vi "GetData.vi"(7 "LabVIEW Web Service Request":refnum<class "Web Request.lvclass">) -> (0 "Ball":T1, 1 "Corners":cluster{"X":sgl, "Y":sgl}[](array[cluster]), 2 "Red Team Data":T2, 3 "Blue Team Data":T2)   [LabVIEW 2018]
uses:
  <vilib>/wsapi/Web Request.lvclass
  Ball Data.vi
  Blue Team Data.vi
  Red Team Data.vi
  Table Data.vi
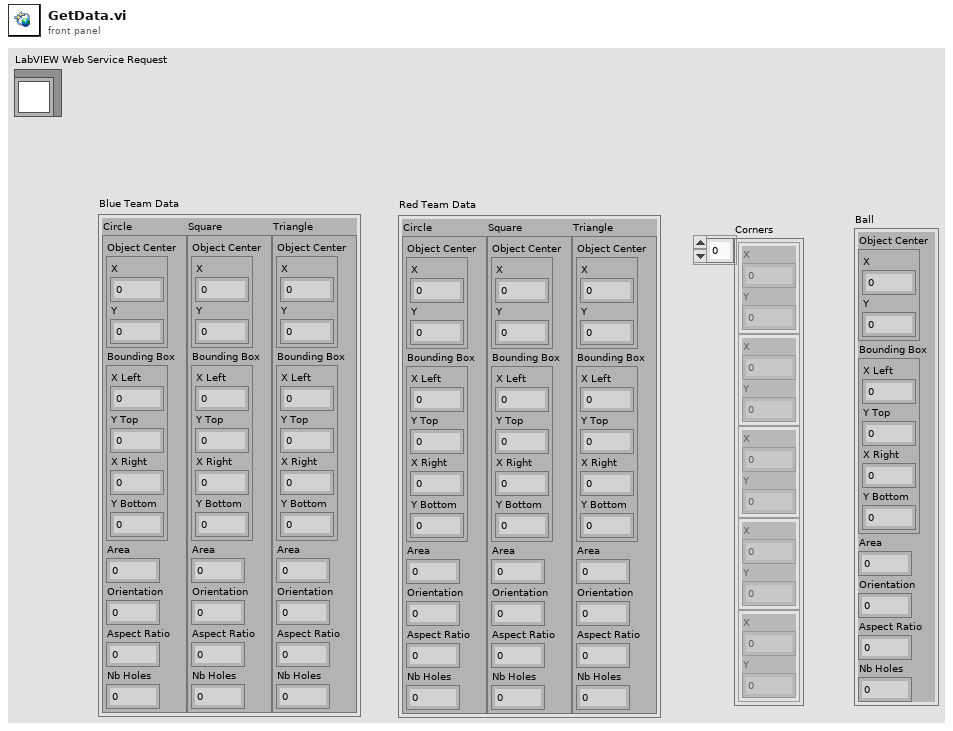
[diagram p1: front panel]
types:
  T1 = cluster{"Object Center":cluster{"X":sgl, "Y":sgl}, "Bounding Box":cluster{"X Left":i32, "Y Top":i32, "X Right":i32, "Y Bottom":i32}, "Area":sgl, "Orientation":sgl, "Aspect Ratio":sgl, "Nb Holes":i32}
  T2 = cluster{"Circle":cluster{"Object Center":cluster{"X":sgl, "Y":sgl}, "Bounding Box":cluster{"X Left":i32, "Y Top":i32, "X Right":i32, "Y Bottom":i32}, "Area":sgl, "Orientation":sgl, "Aspect Ratio":sgl, "Nb Holes":i32}, "Square":cluster{"Object Center":cluster{"X":sgl, "Y":sgl}, "Bounding Box":cluster{"X Left":i32, "Y Top":i32, "X Right":i32, "Y Bottom":i32}, "Area":sgl, "Orientation":sgl, "Aspect Ratio":sgl, "Nb Holes":i32}, "Triangle":cluster{"Object Center":cluster{"X":sgl, "Y":sgl}, "Bounding Box":cluster{"X Left":i32, "Y Top":i32, "X Right":i32, "Y Bottom":i32}, "Area":sgl, "Orientation":sgl, "Aspect Ratio":sgl, "Nb Holes":i32}}
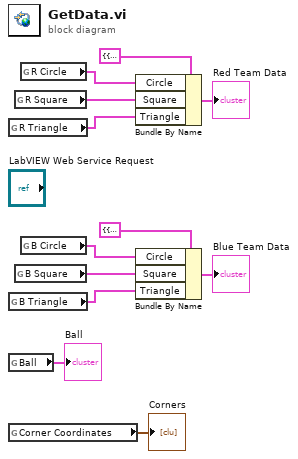
[diagram p0: block diagram]
diagram:
  n1 = global read "Red Team Data.vi" "R Triangle"() -> (w9:T1)
  n2 = global read "Blue Team Data.vi" "B Triangle"() -> (w4:T1)
  n3 = global read "Ball Data.vi" "Ball"() -> (→"Ball":T1)
  n4 = global read "Table Data.vi" "Corner Coordinates"() -> (→"Corners":cluster{"X":sgl, "Y":sgl}[])
  n5 = global read "Red Team Data.vi" "R Square"() -> (w10:T1)
  n6 = global read "Blue Team Data.vi" "B Square"() -> (w5:T1)
  n7 = global read "Red Team Data.vi" "R Circle"() -> (w11:T1)
  n8 = global read "Blue Team Data.vi" "B Circle"() -> (w6:T1)
  n9 = Bundle By Name(cluster=T2 {"Circle"={"Object Center"={"X"=0.0, "Y"=0.0}, "Bounding Box"={"X Left"=0, "Y Top"=0, "X Right"=0, "Y Bottom"=0}, "Area"=0.0, "Orientation"=0.0, "Aspect Ratio"=0.0, "Nb Holes"=0}, "Square"={"Object Center"={"X"=0.0, "Y"=0.0}, "Bounding Box"={"X Left"=0, "Y Top"=0, "X Right"=0, "Y Bottom"=0}, "Area"=0.0, "Orientation"=0.0, "Aspect Ratio"=0.0, "Nb Holes"=0}, "Triangle"={"Object Center"={"X"=0.0, "Y"=0.0}, "Bounding Box"={"X Left"=0, "Y Top"=0, "X Right"=0, "Y Bottom"=0}, "Area"=0.0, "Orientation"=0.0, "Aspect Ratio"=0.0, "Nb Holes"=0}} ("Red Team Data 2"), "Circle"=w11, "Square"=w10, "Triangle"=w9) -> (→"Red Team Data":T2)
  n10 = Bundle By Name(cluster=T2 {"Circle"={"Object Center"={"X"=0.0, "Y"=0.0}, "Bounding Box"={"X Left"=0, "Y Top"=0, "X Right"=0, "Y Bottom"=0}, "Area"=0.0, "Orientation"=0.0, "Aspect Ratio"=0.0, "Nb Holes"=0}, "Square"={"Object Center"={"X"=0.0, "Y"=0.0}, "Bounding Box"={"X Left"=0, "Y Top"=0, "X Right"=0, "Y Bottom"=0}, "Area"=0.0, "Orientation"=0.0, "Aspect Ratio"=0.0, "Nb Holes"=0}, "Triangle"={"Object Center"={"X"=0.0, "Y"=0.0}, "Bounding Box"={"X Left"=0, "Y Top"=0, "X Right"=0, "Y Bottom"=0}, "Area"=0.0, "Orientation"=0.0, "Aspect Ratio"=0.0, "Nb Holes"=0}} ("Blue Team Data 2"), "Circle"=w6, "Square"=w5, "Triangle"=w4) -> (→"Blue Team Data":T2)
